vi "Tusk.Init.vi"(5 "Priority?":bool, 7 "Timeout (ms)(-1)":i32=-1, 8 "error in (no error)":errorcluster, 9 "Data":variant, 11 "Tusk in":refnum<class "Tusk.lvclass">) -> (0 "error out":errorcluster, 1 "Timed out?":bool, 3 "Tusk out":refnum<class "Tusk.lvclass">)   [LabVIEW 2018, in "Application.lvlib" / "Tusk.lvclass"]
uses:
  Tusk.lvclass
  Tusk.lvclass/Tusk.ctl
  Message Class/Message.lvclass/Message.ctl
  Exceptions Class/VIs/Invalid Type.vi
  <vilib>/Utility/error.llb/Trim Whitespace.vi
  Message Class/Message.lvclass
  Keywords Class/Keywords.lvclass
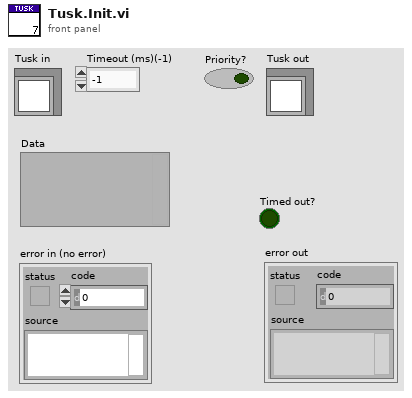
[diagram p1: front panel]
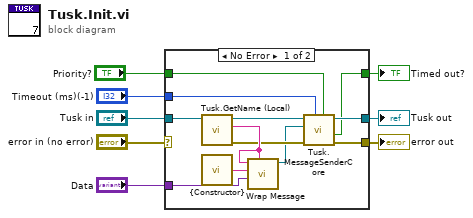
[diagram p0: block diagram]
diagram:
  n1 = case shown="No Error" "error in (no error)" {
    selector: "error in (no error)" -> [_ w22]
    tunnel: [w13 w22] -> w7
    tunnel: [w10 w21] -> w5
    tunnel: "Tusk in" -> [w19 w21]
    tunnel: "Data" -> [w17 _]
    tunnel: "Timeout (ms)(-1)" -> [w12 _]
    tunnel: "Priority?" -> [w11 _]
    tunnel: [w9 _] -> w1
    frame No Error {
      n2 = call "Tusk.GetName (Local).vi"("Tusk in"=w19) -> ("error out"=w16:errorcluster, "Name(Local)"=w18:string, "Tusk out"=w15:refnum<class "Tusk.lvclass">)  [unwired: 8 in]
      n3 = call "{Constructor}.vi"() -> ("Word"=w20:string)  [unwired: 6 in]
      n4 = call "Wrap Message.vi"("Sender"=w18, "Data"=w17, "Message"=w20, "Recipient"=w18) -> ("Message out"=w14:refnum<class "Message.lvclass">)  [unwired: 6 in, 1 out]
      n5 = call "Tusk.MessageSenderCore.vi"("Priority?"=w11, "Timeout (ms)(-1)"=w12, "error in (no error)"=w16, "Message"=w14, "Tusk in"=w15) -> ("error out"=w13:errorcluster, "Timed out?"=w9:bool, "Tusk out"=w10:refnum<class "Tusk.lvclass">)  [unwired: 4 in]
    }
    frame Error {
    }
  }
  "error out" <- w7
  "Tusk out" <- w5
  "Timed out?" <- w1
